vi "Read Waveform.vi"   [LabVIEW 2020, in "Template - Scope.lvlib"]
doc: "Allows users to read one or more waveforms from the oscilloscope."
uses:
  <instrlib>/_Template - Scope/Template - Scope.lvlib
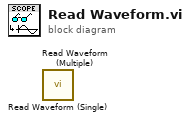
[diagram p0: block diagram]
diagram:
  n1 = call <instrlib>:"Read Waveform (Single).vi"() -> ()  [unwired: 9 in, 3 out]
  n2 = call <instrlib>:"Read Waveform (Multiple).vi"() -> ()  [unwired: 9 in, 3 out]
